vi "test.vi"() -> ()   [LabVIEW 2016]
panel:
  in  "input 1":u32
  out "bytes written":i32
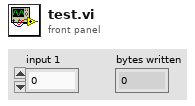
[diagram p1: front panel]
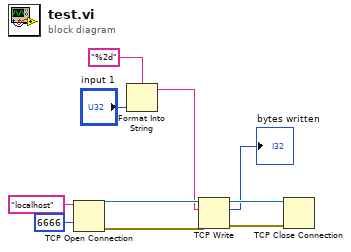
[diagram p0: block diagram]
diagram:
  n1 = TCP Open Connection(address="localhost", remote port or service name=u16 6666) -> (connection ID=w8:refnum<k5>, error out=w7:errorcluster)  [unwired: 3 in]
  n2 = Format Into String(format string="%2d", "input 1") -> (resulting string=w2:string)  [unwired: 2 in, 1 out]
  n3 = TCP Write(connection ID=w8, data in=w2, error in (no error)=w7) -> (connection ID out=w6:refnum<k5>, bytes written=→"bytes written":i32, error out=w5:errorcluster)  [unwired: 1 in]
  n4 = TCP Close Connection(connection ID=w6, error in (no error)=w5) -> ()  [unwired: 1 in, 2 out]
